vi "DT_Check In Circle.vi"(8 "p 4":cluster{"x":dbl, "y":dbl, "index":i32}, 9 "p 3":cluster{"x":dbl, "y":dbl, "index":i32}, 10 "p 2":cluster{"x":dbl, "y":dbl, "index":i32}, 11 "p 1":cluster{"x":dbl, "y":dbl, "index":i32}) -> (3 "in circle?":bool)   [LabVIEW 2020, in "NI_AAL_Geometry.lvlib"]
uses:
  <vilib>/Analysis/NI_AAL_Geometry.lvlib
  <vilib>/Analysis/baseanly.llb/Real Determinant.vi
  <vilib>/Analysis/NI_AALBase.lvlib
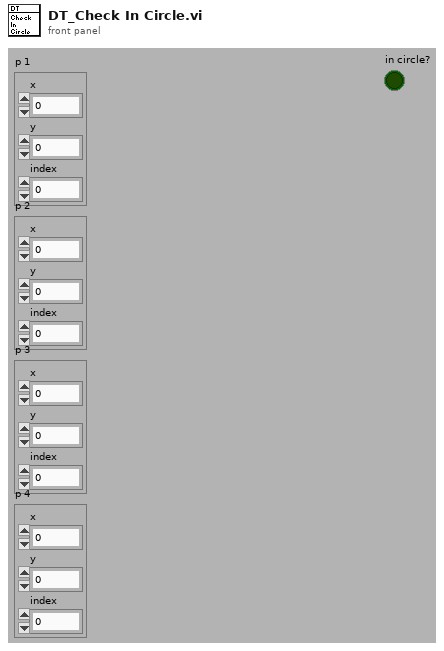
[diagram p1: front panel]
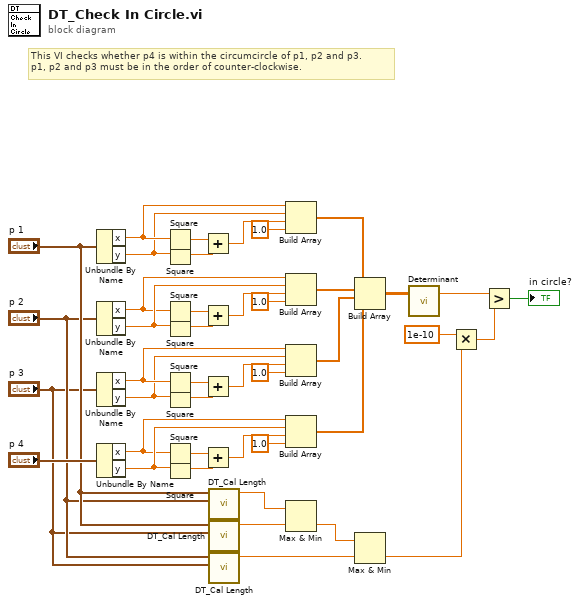
[diagram p0: block diagram]
diagram:
  # "This VI checks whether p4 is within the circumcircle of p1, p2 and p3.\np1, p2 and p3 must be in the order of counter-clockwise."
  n1 = Unbundle By Name("p 1") -> ("x"=w40:dbl, "y"=w39:dbl)
  n2 = Unbundle By Name("p 2") -> ("x"=w33:dbl, "y"=w34:dbl)
  n3 = Unbundle By Name("p 3") -> ("x"=w28:dbl, "y"=w27:dbl)
  n4 = Unbundle By Name("p 4") -> ("x"=w21:dbl, "y"=w22:dbl)
  n5 = Square(x=w40) -> (x^2=w42:dbl)
  n6 = Square(x=w39) -> (x^2=w41:dbl)
  n7 = Square(x=w33) -> (x^2=w31:dbl)
  n8 = Square(x=w34) -> (x^2=w32:dbl)
  n9 = Square(x=w28) -> (x^2=w30:dbl)
  n10 = Square(x=w27) -> (x^2=w29:dbl)
  n11 = Square(x=w21) -> (x^2=w19:dbl)
  n12 = Square(x=w22) -> (x^2=w20:dbl)
  n13 = Add(x=w42, y=w41) -> (x+y=w38:dbl)
  n14 = Add(x=w31, y=w32) -> (x+y=w35:dbl)
  n15 = Add(x=w30, y=w29) -> (x+y=w26:dbl)
  n16 = Add(x=w19, y=w20) -> (x+y=w23:dbl)
  n17 = call <vilib>:"DT_Cal Length.vi"("p 2"="p 2", "p 1"="p 1") -> ("length"=w4:dbl)  [unwired: 9 out]
  n18 = call <vilib>:"DT_Cal Length.vi"("p 2"="p 3", "p 1"="p 1") -> ("length"=w3:dbl)  [unwired: 9 out]
  n19 = call <vilib>:"DT_Cal Length.vi"("p 2"="p 3", "p 1"="p 2") -> ("length"=w1:dbl)  [unwired: 9 out]
  n20 = Build Array(w40, w39, w38, 1.0 ("element")) -> (w17:dbl[])
  n21 = Build Array(w33, w34, w35, 1.0 ("element")) -> (w16:dbl[])
  n22 = Build Array(w28, w27, w26, 1.0 ("element")) -> (w15:dbl[])
  n23 = Build Array(w21, w22, w23, 1.0 ("element")) -> (w14:dbl[])
  n24 = Max & Min(x=w4, y=w3) -> (min(x,y)=w2:dbl)  [unwired: 1 out]
  n25 = Build Array(w17, w16, w15, w14) -> (w11:dbl[][])
  n26 = Max & Min(x=w2, y=w1) -> (min(x,y)=w5:dbl)  [unwired: 1 out]
  n27 = call-poly <vilib>:"Determinant.vi"("Input Matrix"=w11) -> ("determinant"=w13:dbl)  [unwired: 1 in, 1 out]
  n28 = Multiply(x=1e-10 ("y"), y=w5) -> (x*y=w9:dbl)
  n29 = Greater?(x=w13, y=w9) -> (0:→"in circle?":bool)
